vi "Programmatically Dig a Grave.vi"() -> ()   [LabVIEW 2017]
doc: "A demonstration of programmatically digging a grave in a VI's block diagram using the Eulogy Toolkit API. The grave is dug in the block diagram for the Dig a Grave - Simple.vi example."
uses:
  <vilib>/Utility/traverseref.llb/TRef TravTarget.ctl
  Toolkit VIs/Toolkit.lvlib
  <vilib>/Utility/traverseref.llb/VI Scripting - Traverse.lvlib
panel:
  in  "Stop Button":bool
  # "Overview: Demonstrates programmatically digging a grave using the Dig a Grave - Simple.vi as a target\nInstructions:\n1. Run the VI\n2. The Dig a Grave - Simple.vi's block diagram will be displayed\n3. A grave will be dug within the box as indicated on the block diagram of the Dig a Grave - Simple.vi example.\n4. Click the Stop button\n5. The programmatic grave digging will be undone to leave the Dig a Grave - Simple.vi example in its original state."
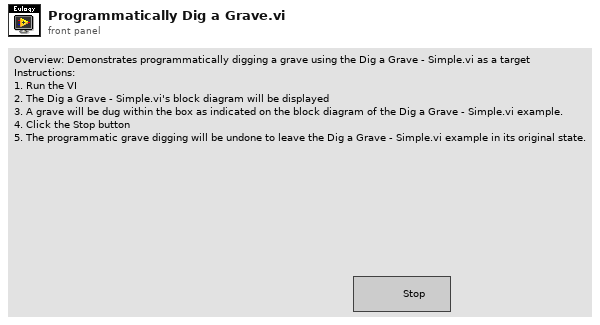
[diagram p1: front panel]
types:
  T1 = typedef "TRef TravTarget.ctl" = enum16{"FP", "BD", "Other"}
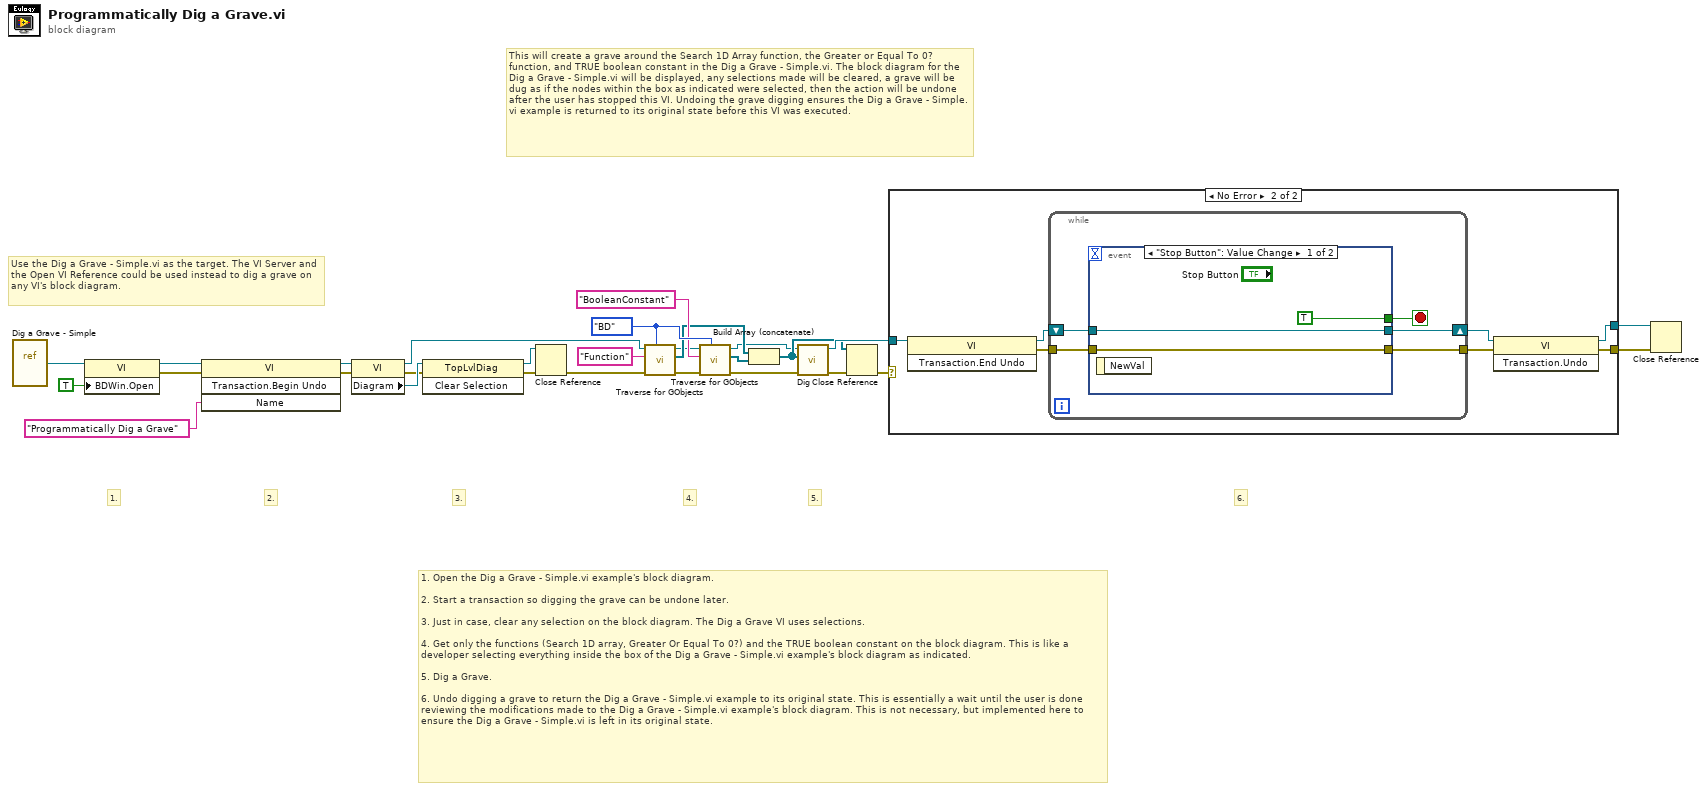
[diagram p0: block diagram]
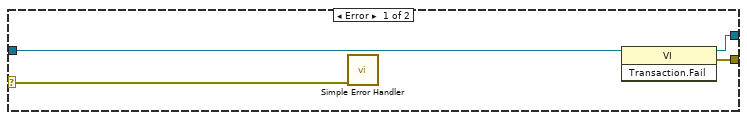
[diagram p2: hidden frame]
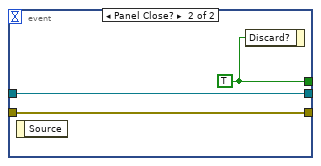
[diagram p3: hidden frame]
diagram:
  w16 = TRef_TravTarget."BD" ("Traverse Target")
  # "This will create a grave around the Search 1D Array function, the Greater or Equal To 0? function, and TRUE boolean constant in the Dig a Grave - Simple.vi. The block diagram for the Dig a Grave - Simple.vi will be displayed, any selections made will be cleared, a grave will be dug as if the nodes within the box as indicated were selected, then the action will be undone after the user has stopped this VI. Undoing the grave digging ensures the Dig a Grave - Simple.vi example is returned to its original state before this VI was executed."
  # "6."
  # "Use the Dig a Grave - Simple.vi as the target. The VI Server and the Open VI Reference could be used instead to dig a grave on any VI's block diagram."
  # "1. Open the Dig a Grave - Simple.vi example's block diagram.\n\n2. Start a transaction so digging the grave can be undone later.\n\n3. Just in case, clear any selection on the block diagram. The Dig a Grave VI uses selections.\n\n4. Get only the functions (Search 1D array, Greater Or Equal To 0?) and the TRUE boolean constant on the block diagram. This is like a developer selecting everything inside the box of the Dig a Grave - Simple.vi example's block diagram as indicated.\n\n5. Dig a Grave.\n\n6. Undo digging a grave to return the Dig a Grave - Simple.vi example to its original state. This is essentially a wait until the user is done reviewing the modifications made to the Dig a Grave - Simple.vi example's block diagram. This is not necessary, but implemented here to ensure the Dig a Grave - Simple.vi is left in its original state."
  # "5."
  # "4."
  # "3."
  # "2."
  # "1."
  n1 = vi-ref "Dig a Grave - Simple.vi"() -> (w21:refnum<vi>)
  n2 = property class="VI"(reference=w21, "BDWin.Open"=TRUE ("Block Diagram Window:Open")) -> (reference out=w20:refnum<vi>, error out=w18:errorcluster)  [unwired: 1 in]
  n3 = invoke class="VI" method="Transaction.Begin Undo"(reference=w20, error in=w18, "Name"="Programmatically Dig a Grave") -> (reference out=w8:refnum<vi>, error out=w7:errorcluster)  [unwired: 1 in, 2 out]
  n4 = property class="VI"(reference=w8, error in=w7) -> (reference out=w2:refnum<vi>, error out=w5:errorcluster, "Diagram"=w6:refnum<vi>)
  n5 = invoke class="TopLvlDiag" method="Clear Selection"(reference=w6, error in=w5) -> (reference out=w3:refnum<vi>, error out=w4:errorcluster)  [unwired: 1 in, 1 out]
  n6 = Close Reference(reference=w3, error in (no error)=w4) -> (error out=w1:errorcluster)
  n7 = call <vilib>:"Traverse for GObjects.vi"("Traverse Target"=w16, "error in (no error)"=w1, "Class Name"="Function", "VI Refnum"=w2) -> ("error out"=w17:errorcluster, "References"=w14:refnum<vi>[], "dup VI Refnum"=w10:refnum<vi>)  [unwired: 4 in, 1 out]
  n8 = call <vilib>:"Traverse for GObjects.vi"("Traverse Target"=w16, "error in (no error)"=w17, "Class Name"="BooleanConstant", "VI Refnum"=w10) -> ("error out"=w11:errorcluster, "References"=w13:refnum<vi>[], "dup VI Refnum"=w9:refnum<vi>)  [unwired: 4 in, 1 out]
  n9 = Build Array (concatenate)(w14, w13) -> (w12:refnum<vi>[])
  n10 = call "Dig.vi"("Error In"=w11, "Selection List[]"=w12, "VI In"=w9) -> ("Error Out"=w24:errorcluster, "VI Out"=w26:refnum<vi>)  [unwired: 7 in]
  n11 = Close Reference(reference=w12, error in (no error)=w24) -> (error out=w22:errorcluster)
  n12 = case shown="No Error" w22 {
    selector: w22 -> [w29 _]
    tunnel: [w32 w35] -> w25
    tunnel: w26 -> [w31 w39]
    tunnel: [w30 w36] -> w23
    frame Error {
      n13 = call <vilib>:"Simple Error Handler.vi"("error in (no error)"=w29) -> ()  [unwired: 4 in, 5 out]
      n14 = invoke class="VI" method="Transaction.Fail"(reference=w31) -> (reference out=w30:refnum<vi>, error out=w32:errorcluster)  [unwired: 2 in, 1 out]
    }
    frame No Error {
      n15 = invoke class="VI" method="Transaction.End Undo"(reference=w39) -> (reference out=w38:refnum<vi>, error out=w34:errorcluster)  [unwired: 2 in, 1 out]
      n16 = while {
        shift-right: [w43] -> w37
        shift-left: w38 -> [w44]
        tunnel: w34 -> [w42]
        tunnel: [w41] -> w33
        stop <- w40 stop-if-true
        n17 = event shown="[0] \"Stop Button\": Value Change" {
          selector: _ -> [_ _]
          dyn-events: _ -> [_ _]
          timeout: _ -> [_ _]
          tunnel: w44 -> [w47 w50]
          tunnel: [w47 w50] -> w43
          tunnel: w42 -> [w46 w49]
          tunnel: [w46 w49] -> w41
          tunnel: [TRUE w48] -> w40
          event "Stop Button": Value Change {
            n18 = event-data() -> ()  [unwired: 1 in, 1 out]
          }
          event Panel Close? {
            w48 = TRUE
            n19 = event-data() -> ()  [unwired: 1 in, 1 out]
            n20 = event-data("Discard?"=w48) -> ()  [unwired: 1 in, 1 out]
          }
        }
      }
      n21 = invoke class="VI" method="Transaction.Undo"(reference=w37, error in=w33) -> (reference out=w36:refnum<vi>, error out=w35:errorcluster)  [unwired: 1 in, 1 out]
    }
  }
  n22 = Close Reference(reference=w23, error in (no error)=w25) -> ()  [unwired: 1 out]
